vi "Update Active Graphic Sytle.vi"(8 "error in (no error)":errorcluster, 10 "Style":T1={"Color"=0, "Pen"={"Width"=2, "Style"=enum."Solid"}}, 11 "Canvas in":refnum<class "Canvas.lvclass">) -> (0 "error out":errorcluster, 3 "Canvas out":refnum<class "Canvas.lvclass">)   [LabVIEW 2015, in "Canvas.lvclass"]
uses:
  Canvas.lvclass
  Graphic/Ctls/Style.ctl
  Canvas.lvclass/Canvas.ctl
  Graphic/Graphic.lvclass/Graphic.ctl
  Graphic/Graphic.lvclass
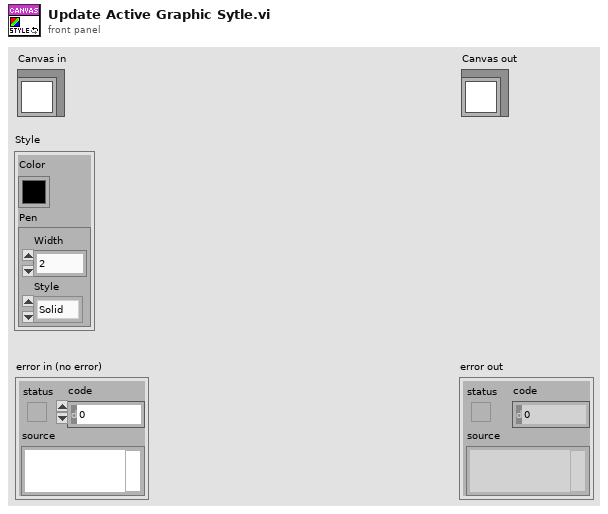
[diagram p1: front panel]
types:
  T1 = typedef "Graphic.lvclass/Style.ctl" = cluster{"Color":u32, "Pen":cluster{"Width":u16, "Style":enum32{"Solid", "Dash", "Dot", "DashDot", "DashDotDot"}}}
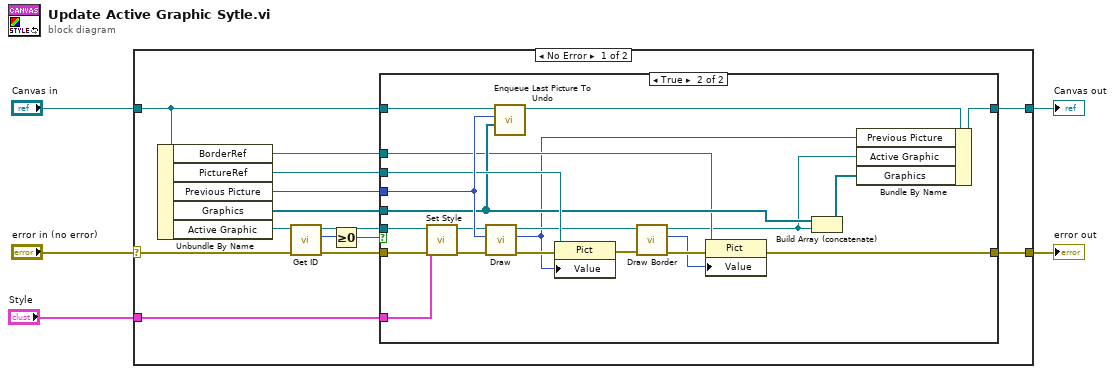
[diagram p0: block diagram]
diagram:
  n1 = case shown="No Error" "error in (no error)" {
    selector: "error in (no error)" -> [w9 w44]
    tunnel: [w14 w44] -> w4
    tunnel: [w15 w43] -> w2
    tunnel: "Canvas in" -> [w19 w43]
    tunnel: "Style" -> [w13 _]
    frame No Error {
      n2 = Unbundle By Name(w19) -> ("BorderRef"=w12:refnum<vi>, "PictureRef"=w17:refnum<vi>, "Previous Picture"=w18:picture, "Graphics"=w16:refnum<class "Graphic.lvclass">[], "Active Graphic"=w10:refnum<class "Graphic.lvclass">)
      n3 = call "Get ID.vi"("error in (no error)"=w9, "Graphic in"=w10) -> ("error out"=w7:errorcluster, "ID"=w11:i32, "Graphic out"=w8:refnum<class "Graphic.lvclass">)  [unwired: 7 in]
      n4 = Greater Or Equal To 0?(x=w11) -> (x >= 0?=w6:bool)
      n5 = case shown="True" w6 {
        tunnel: w8 -> [_ w42]
        tunnel: w19 -> [w21 w41]
        tunnel: w18 -> [_ w40]
        tunnel: w17 -> [_ w39]
        tunnel: w16 -> [_ w38]
        tunnel: [w21 w37] -> w15
        tunnel: [w20 w36] -> w14
        tunnel: w7 -> [w20 w35]
        tunnel: w13 -> [_ w34]
        tunnel: w12 -> [_ w33]
        frame False {
        }
        frame True {
          n6 = call "Set Style.vi"("error in (no error)"=w35, "Style"=w34, "Graphic in"=w42) -> ("error out"=w30:errorcluster, "Graphic out"=w32:refnum<class "Graphic.lvclass">)  [unwired: 7 in]
          n7 = call-dynamic "Draw.vi"("error in (no error)"=w30, "Picture in"=w40, "Graphic in"=w32) -> ("error out"=w29:errorcluster, "Picture out"=w24:picture, "Graphic out"=w28:refnum<class "Graphic.lvclass">)  [unwired: 6 in]
          n8 = call "Enqueue Last Picture To Undo.vi"("Graphics"=w38, "Last Picture"=w40, "Canvas in"=w41) -> ("Canvas out"=w31:refnum<class "Canvas.lvclass">)  [unwired: 7 in, 1 out]
          n9 = property class="Pict"(reference=w39, error in=w29, "Value"=w24) -> (error out=w27:errorcluster)  [unwired: 1 out]
          n10 = call-dynamic "Draw Border.vi"("error in (no error)"=w27, "Graphic in"=w28) -> ("error out"=w23:errorcluster, "Picture out"=w22:picture, "Graphic out"=w25:refnum<class "Graphic.lvclass">)  [unwired: 7 in]
          n11 = property class="Pict"(reference=w33, error in=w23, "Value"=w22) -> (error out=w36:errorcluster)  [unwired: 1 out]
          n12 = Build Array (concatenate)(w38, w25) -> (w26:refnum<class "Graphic.lvclass">[])
          n13 = Bundle By Name(cluster=w31, "Previous Picture"=w24, "Active Graphic"=w25, "Graphics"=w26) -> (w37:refnum<class "Canvas.lvclass">)
        }
      }
    }
    frame Error {
    }
  }
  "error out" <- w4
  "Canvas out" <- w2
